vi "HIOKI PW3390 Conf Noise analysis.vi"(0 "VISA Resource":refnum<visa-resource-name>, 1 "Analysis CH (0: CH1)":enum16{"CH1", "CH2", "CH3", "CH4"}(ring), 2 "Sampling (4: 250kS)":T1(ring)=enum."250kS", 3 "Points (2: 10000)":enum16{"1000", "5000", "10000", "50000"}(ring)=enum."10000", 4 "Lowest Noise Freq (1: 1kHz)":T2(ring)=enum."1kHz", 5 "error in (no error)":errorcluster, 6 "Set/Query (F: Set)":bool, 7 "Window Type (1: Hanning)":enum16{"rectangular", "hanning", "flat top"}(ring)=enum."hanning", 9 "OPC query (T: ON)":bool=TRUE, 11 "Error Out (F: Off)":bool) -> (13 "Window Type out":enum16{"rectangular", "hanning", "flat top"}(ring)=enum."hanning", 14 "VISA Resource out":refnum<visa-resource-name>, 15 "Analysis CH out":enum16{"CH1", "CH2", "CH3", "CH4"}(ring), 16 "Sampling out":T1(ring)=enum."250kS", 17 "Points out":i32=10000 min=1 max=6, 18 "Lowest Noise Freq out":T2(ring)=enum."1kHz", 19 "error out":errorcluster)   [LabVIEW 2009]
doc: "Set/Query\n Set: Send the setting commands for the device.\n Query: Query the setting of the device.\n\nLowest Noise Freq\n Sets the noise lowest frequency.\n\nPoints\n Sets the point value for Noise Analysis.\n\nSampling\n Sets the sampling speed for Noise Analysis. \n\nWindow Type\n Sets the Noise Analysis Window Function.\n\n<B>Note</B>\nThe lowest noise frequency may be restricted depending on the setting of the noise analysis sampling speed."
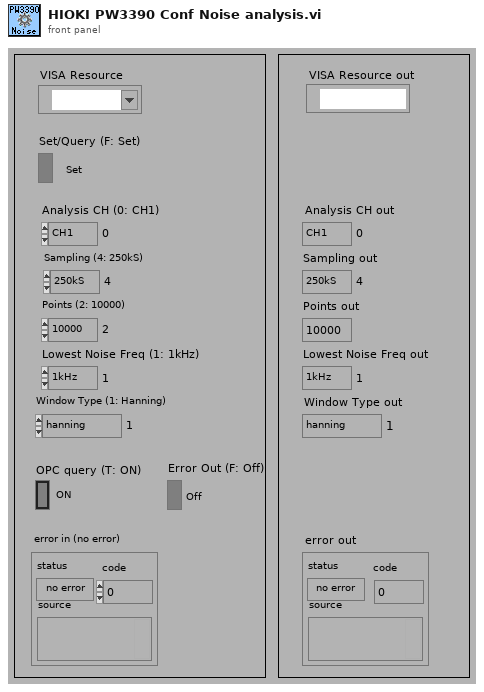
[diagram p1: front panel]
types:
  T1 = enum16{"10kS", "25kS", "50kS", "100kS", "250kS", "500kS"}
  T2 = enum16{"OFF", "1kHz", "2kHz", "3kHz", "4kHz", "5kHz", "6kHz", "7kHz", "8kHz", "9kHz", "10kHz"}
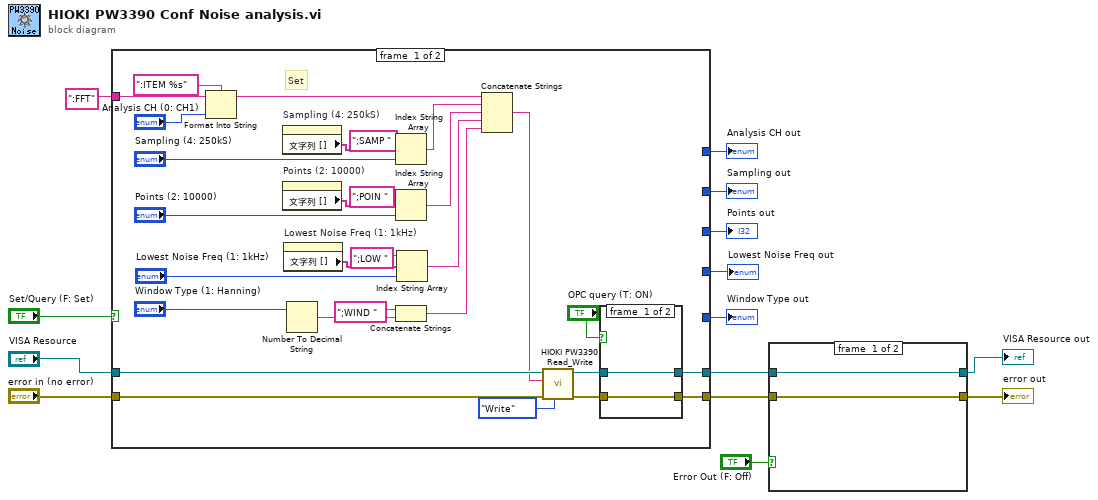
[diagram p0: block diagram]
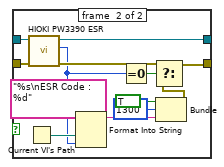
[diagram p2: hidden frame]
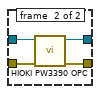
[diagram p3: hidden frame]
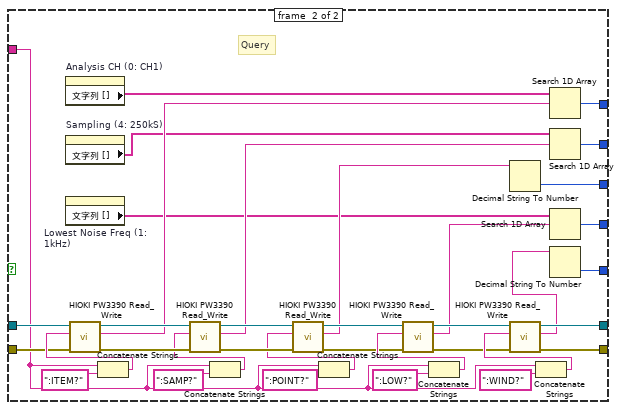
[diagram p4: hidden frame]
diagram:
  n1 = case shown="TRUE" "Set/Query (F: Set)" {
    tunnel: "error in (no error)" -> [w41 w80]
    tunnel: [w20 w65] -> w11
    tunnel: "VISA Resource" -> [w42 w82]
    tunnel: [w21 w64] -> w10
    tunnel: ":FFT" -> [w39 w63]
    tunnel: [_ w53] -> w6
    tunnel: [_ w54] -> w7
    tunnel: [_ w62] -> w2
    tunnel: [_ w59] -> w1
    tunnel: [_ w58] -> w5
    frame #0 {
      # "Set"
      n2 = Format Into String(format string=":ITEM %s" ("形式文字列"), initial string=w39, "Analysis CH (0: CH1)") -> (resulting string=w30:string)  [unwired: 1 in, 1 out]
      n3 = property on="Sampling (4: 250kS)" class="Enum (strict)"() -> ("文字列 []"=w37:string[])  [unwired: 2 in, 2 out]
      n4 = property on="Points (2: 10000)" class="Enum (strict)"() -> ("文字列 []"=w36:string[])  [unwired: 2 in, 2 out]
      n5 = property on="Lowest Noise Freq (1: 1kHz)" class="Enum (strict)"() -> ("文字列 []"=w17:string[])  [unwired: 2 in, 2 out]
      n6 = Number To Decimal String(number="Window Type (1: Hanning)") -> (decimal integer string=w26:string)  [unwired: 1 in]
      n7 = Index String Array(1:"Sampling (4: 250kS)", 2:w37, 3:";SAMP ") -> (0:w16:string)
      n8 = Index String Array(1:"Points (2: 10000)", 2:w36, 3:";POIN ") -> (0:w29:string)
      n9 = Concatenate Strings(";WIND " ("文字列"), w26) -> (w27:string)
      n10 = Index String Array(1:"Lowest Noise Freq (1: 1kHz)", 2:w17, 3:";LOW ") -> (0:w15:string)
      n11 = Concatenate Strings(w30, w16, w29, w15, w27) -> (w28:string)
      n12 = call <instrlib>:"HIOKI PW3390 Read_Write.vi"("Read/Write"=enum16{"Read", "Write"}."Write", "error in (no error)"=w41, "data in"=w28, "VISA Resource"=w42) -> ("error out"=w22:errorcluster, "VISA Resource out"=w23:refnum<visa-resource-name>)  [unwired: 5 in, 1 out]
      n13 = case shown="TRUE" "OPC query (T: ON)" {
        tunnel: [w45 w49] -> w21
        tunnel: [w44 w48] -> w20
        tunnel: w23 -> [w45 w47]
        tunnel: w22 -> [w44 w46]
        frame #0 {
        }
        frame #1 {
          n14 = call <instrlib>:"HIOKI PW3390 OPC.vi"("error in (no error)"=w46, "VISA Resource"=w47) -> ("error out"=w48:errorcluster, "VISA Resource out"=w49:refnum<visa-resource-name>)  [unwired: 7 in, 1 out]
        }
      }
    }
    frame #1 {
      # "Query"
      n15 = property on="Analysis CH (0: CH1)" class="Enum (strict)"() -> ("文字列 []"=w55:string[])  [unwired: 2 in, 2 out]
      n16 = property on="Sampling (4: 250kS)" class="Enum (strict)"() -> ("文字列 []"=w51:string[])  [unwired: 2 in, 2 out]
      n17 = property on="Lowest Noise Freq (1: 1kHz)" class="Enum (strict)"() -> ("文字列 []"=w50:string[])  [unwired: 2 in, 2 out]
      n18 = Concatenate Strings(w63, ":ITEM?") -> (w81:string)
      n19 = call <instrlib>:"HIOKI PW3390 Read_Write.vi"("error in (no error)"=w80, "data in"=w81, "VISA Resource"=w82) -> ("error out"=w78:errorcluster, "data out"=w56:string, "VISA Resource out"=w79:refnum<visa-resource-name>)  [unwired: 6 in]
      n20 = Concatenate Strings(w63, ":SAMP?") -> (w77:string)
      n21 = call <instrlib>:"HIOKI PW3390 Read_Write.vi"("error in (no error)"=w78, "data in"=w77, "VISA Resource"=w79) -> ("error out"=w75:errorcluster, "data out"=w61:string, "VISA Resource out"=w76:refnum<visa-resource-name>)  [unwired: 6 in]
      n22 = Concatenate Strings(w63, ":POINT?") -> (w74:string)
      n23 = call <instrlib>:"HIOKI PW3390 Read_Write.vi"("error in (no error)"=w75, "data in"=w74, "VISA Resource"=w76) -> ("error out"=w71:errorcluster, "data out"=w52:string, "VISA Resource out"=w70:refnum<visa-resource-name>)  [unwired: 6 in]
      n24 = Concatenate Strings(w63, ":LOW?") -> (w73:string)
      n25 = call <instrlib>:"HIOKI PW3390 Read_Write.vi"("error in (no error)"=w71, "data in"=w73, "VISA Resource"=w70) -> ("error out"=w66:errorcluster, "data out"=w60:string, "VISA Resource out"=w67:refnum<visa-resource-name>)  [unwired: 6 in]
      n26 = Decimal String To Number(string=w52) -> (number=w53:i32)  [unwired: 2 in, 1 out]
      n27 = Concatenate Strings(w63, ":WIND?") -> (w68:string)
      n28 = call <instrlib>:"HIOKI PW3390 Read_Write.vi"("error in (no error)"=w66, "data in"=w68, "VISA Resource"=w67) -> ("error out"=w65:errorcluster, "data out"=w57:string, "VISA Resource out"=w64:refnum<visa-resource-name>)  [unwired: 6 in]
      n29 = Search 1D Array(1D array=w55, element=w56) -> (index of element=w54:i32)  [unwired: 1 in]
      n30 = Search 1D Array(1D array=w51, element=w61) -> (index of element=w62:i32)  [unwired: 1 in]
      n31 = Search 1D Array(1D array=w50, element=w60) -> (index of element=w59:i32)  [unwired: 1 in]
      n32 = Decimal String To Number(string=w57) -> (number=w58:i32)  [unwired: 2 in, 1 out]
    }
  }
  "Lowest Noise Freq out" <- w1
  "Analysis CH out" <- w7
  "Points out" <- w6
  "Sampling out" <- w2
  "Window Type out" <- w5
  n33 = case shown="TRUE" "Error Out (F: Off)" {
    tunnel: w10 -> [w87 w100]
    tunnel: w11 -> [w86 w99]
    tunnel: [w86 w89] -> w9
    tunnel: [w87 w98] -> w3
    frame #0 {
    }
    frame #1 {
      n34 = Current VI's Path() -> (path=w96:path)
      n35 = call <instrlib>:"HIOKI PW3390 ESR.vi"("error in (no error)"=w99, "VISA Resource"=w100) -> ("error out"=w90:errorcluster, "Output Value"=w88:u8, "VISA Resource out"=w98:refnum<visa-resource-name>)  [unwired: 6 in, 1 out]
      n36 = Format Into String(format string="%s\nESR Code : %d", w96, w88) -> (resulting string=w92:string)  [unwired: 2 in, 1 out]
      n37 = Equal To 0?(x=w88) -> (x = 0?=w97:bool)
      n38 = Bundle("status"=TRUE, "code"=1300, w92) -> (w91:cluster{"status":bool, "code":i32, string})  [unwired: 1 in]
      n39 = Select(t=w90, s=w97, f=w91) -> (s? t:f=w89:errorcluster)
    }
  }
  "error out" <- w9
  "VISA Resource out" <- w3
